vi "Set Capillary Valve Interlock Configuration.vi"(8 "error in (no error)":errorcluster, 9 "Manual Mode (False)":bool, 10 "Open? (False)":bool, 11 "Capillary Line in":refnum<class "Capillary Line.lvclass">) -> (0 "error out":errorcluster, 1 "Interlock Chain":refnum<class "Interlock Chain.lvclass">, 2 "Open? (False)":bool, 3 "Capillary Line out":refnum<class "Capillary Line.lvclass">)   [LabVIEW 2015, in "cRIO-Carbondioxide.lvlib" / "CO2-Actor.lvlib" / "Capillary Line.lvclass"]
uses:
  Capillary Line.lvclass
  Interlocks/Interlock Chain/Interlock Chain.lvclass
  Interlocks/Interlock/Interlock.lvclass
  Controls/Sample Push State Enumerator.ctl
  Interlocks/Controls/Add IL to -Enumerator.ctl
  Interlocks/Interlock Bool/Interlock Bool.lvclass
  Interlocks/Interlock Bool/Interlock Bool.lvclass/Interlock Bool.ctl
  Interlocks/Interlock Chain/Interlock Chain.lvclass/Interlock Chain.ctl
  cRIO-CO2/cRIO-CO2.lvclass
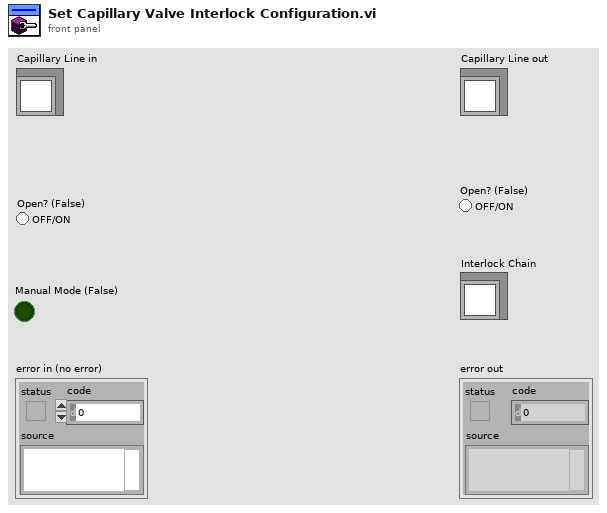
[diagram p1: front panel]
types:
  T1 = typedef "Add IL to -Enumerator.ctl" = enum16{"Deny", "Allow", "None"}
  T2 = typedef "Sample Push State Enumerator.ctl" = enum16{"Undefined", "Initialize", "Dilute", "Close Transfer Line", "Start Heaters", "Warm Up Syringe", "Ready to Push", "Push", "Initiate Stash", "Stash", "Complete", "Abort", "Idle", "Error"}
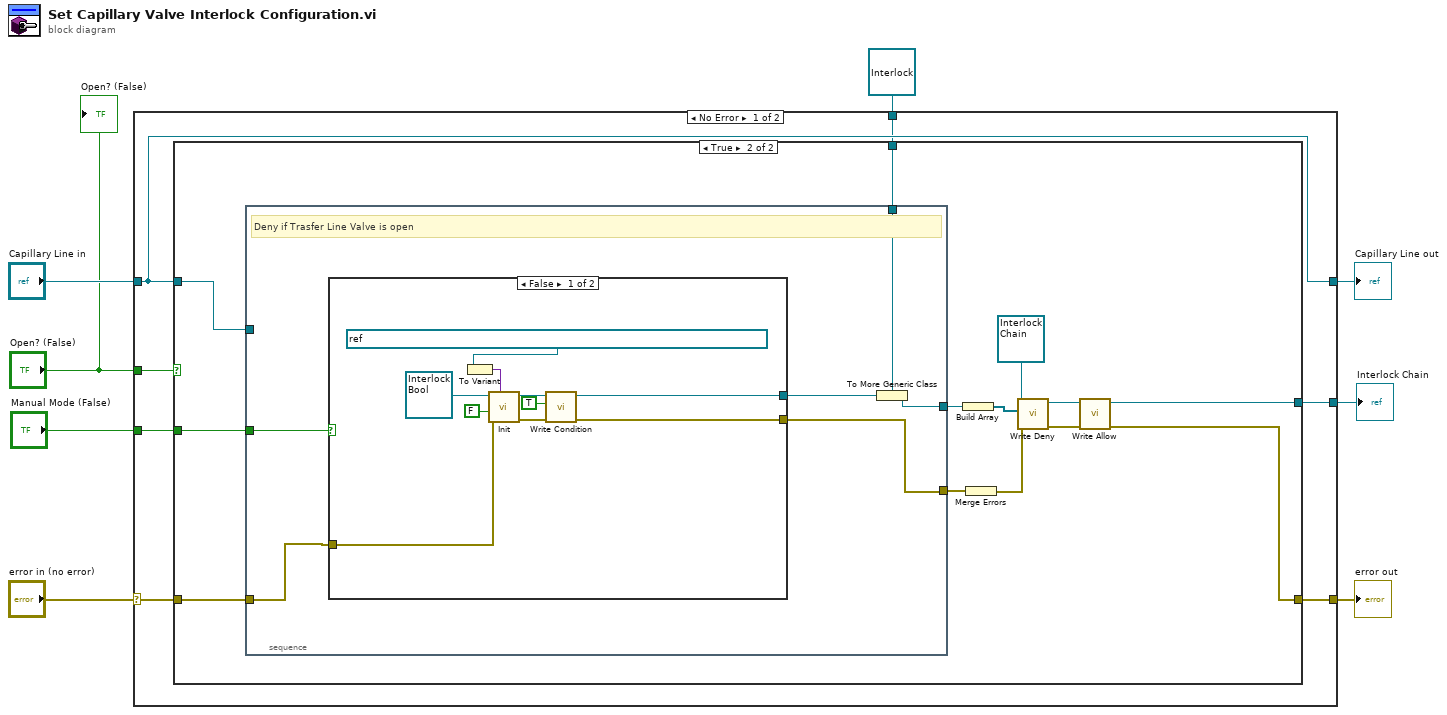
[diagram p0: block diagram]
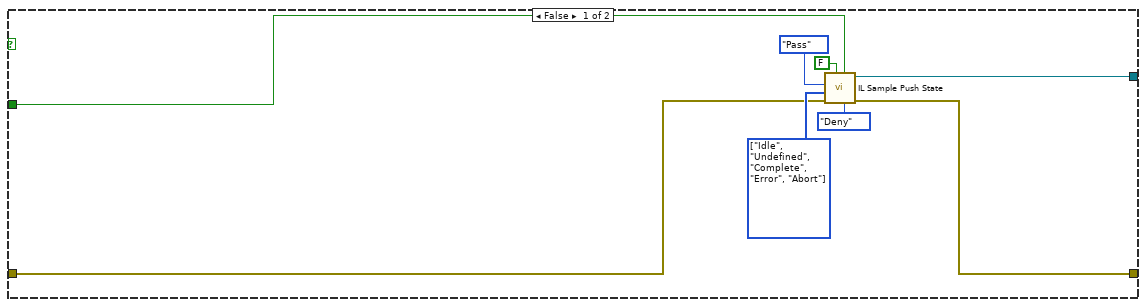
[diagram p2: hidden frame]
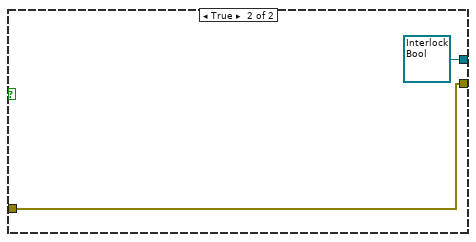
[diagram p3: hidden frame]
diagram:
  n1 = case shown="No Error" "error in (no error)" {
    selector: "error in (no error)" -> [w14 w56]
    tunnel: [w12 w56] -> w7
    tunnel: [w11 w55] -> w5
    tunnel: "Capillary Line in" -> [w11 w55]
    tunnel: "Manual Mode (False)" -> [w15 _]
    tunnel: [w13 _] -> w3
    tunnel: refnum<class "Interlock.lvclass"> refnum ("Interlock.lvclass") -> [w10 _]
    tunnel: "Open? (False)" -> [w9 _]
    frame No Error {
      n2 = case shown="True" w9 {
        tunnel: w15 -> [w17 w36]
        tunnel: w14 -> [w20 w35]
        tunnel: [w18 w25] -> w13
        tunnel: [w19 w24] -> w12
        tunnel: w11 -> [_ w30]
        tunnel: w10 -> [_ w29]
        frame False {
          w21 = T2[] [enum."Idle", enum."Undefined", enum."Complete", enum."Error", enum."Abort"] items=["Undefined", "Initialize", "Dilute", "Close Transfer Line", "Start Heaters", "Warm Up Syringe", "Ready to Push", "Push", "Initiate Stash", "Stash", "Complete", "Abort", "Idle", "Error"] ("States")
          n3 = call "IL Sample Push State.vi"("Add to (Deny)"=Add_IL_to_-Enumerator."Deny", "Ignore (F)"=w17, "Stop Self on IL? (T)"=FALSE, "error in (no error)"=w20, "States"=w21, "Pass/Seize"=enum16{"Pass", "Seize"}."Pass") -> ("error out"=w19:errorcluster, "Interlock Chain out"=w18:refnum<class "Interlock Chain.lvclass">)  [unwired: 3 in, 1 out]
        }
        frame True {
          n4 = stacked-sequence {
            tunnel: w36 -> [w42]
            tunnel: w30 -> [_]
            tunnel: w35 -> [w37]
            tunnel: w29 -> [w40]
            tunnel: [w41] -> w28
            tunnel: [w38] -> w27
            frame #0 {
              # "Deny if Trasfer Line Valve is open"
              n5 = case shown="False" w42 {
                tunnel: [w46 w53] -> w41
                tunnel: [w45 refnum<class "Interlock Bool.lvclass"> refnum ("Interlock Bool out")] -> w39
                tunnel: w37 -> [w44 w53]
                frame False {
                  n6 = To Variant(anything=refnum<k21> "ni.var.psp://crio-carbondioxide/AMS Gas SHV/Valves/Syringe-Line Valve HV314" ("shared variable refnum in")) -> (Variant=w50:variant)
                  n7 = call-dynamic "Init.vi"("SHV"=w50, "error in (no error)"=w44, "Stop Self on IL? (T)"=FALSE, "Interlock in"=refnum<class "Interlock Bool.lvclass"> refnum ("Interlock Bool.lvclass")) -> ("error out"=w49:errorcluster, "Interlock out"=w48:refnum<class "Interlock Bool.lvclass">)  [unwired: 6 in]
                  n8 = call "Write Condition.vi"("error in (no error)"=w49, "Interlock Condition"=TRUE, "Interlock Bool in"=w48) -> ("error out"=w46:errorcluster, "Interlock Bool out"=w45:refnum<class "Interlock Bool.lvclass">)  [unwired: 7 in]
                }
                frame True {
                }
              }
              n9 = To More Generic Class(target class=w40, reference=w39) -> (generic class reference=w38:refnum<class "Interlock.lvclass">)
            }
          }
          n10 = Build Array(w27) -> (w26:refnum<class "Interlock.lvclass">[])
          n11 = Merge Errors(w28) -> (w32:errorcluster)
          n12 = call "Write Deny.vi"("error in (no error)"=w32, "Deny"=w26, "Interlock Chain in"=refnum<class "Interlock Chain.lvclass"> refnum) -> ("error out"=w31:errorcluster, "Interlock Chain out"=w34:refnum<class "Interlock Chain.lvclass">)  [unwired: 7 in]
          n13 = call "Write Allow.vi"("error in (no error)"=w31, "Interlock Chain in"=w34) -> ("error out"=w24:errorcluster, "Interlock Chain out"=w25:refnum<class "Interlock Chain.lvclass">)  [unwired: 8 in]
        }
      }
    }
    frame Error {
    }
  }
  "error out" <- w7
  "Capillary Line out" <- w5
  "Interlock Chain" <- w3
  "Open? (False)" <- "Open? (False)"
